vi "Fit and Plot Metric v2.vi"() -> (3 "Peak":dbl)   [LabVIEW 2014]
uses:
  <vilib>/Analysis/NI_AALPro.lvlib
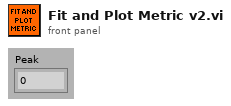
[diagram p1: front panel]
types:
  T1 = cluster{"Ab Corr VI.I":dbl[], "Ab Corr VI.I":dbl[]}
  T2 = cluster{"Ab Corr VI.I":dbl[], "Ab Corr VI.I":dbl[]}[]
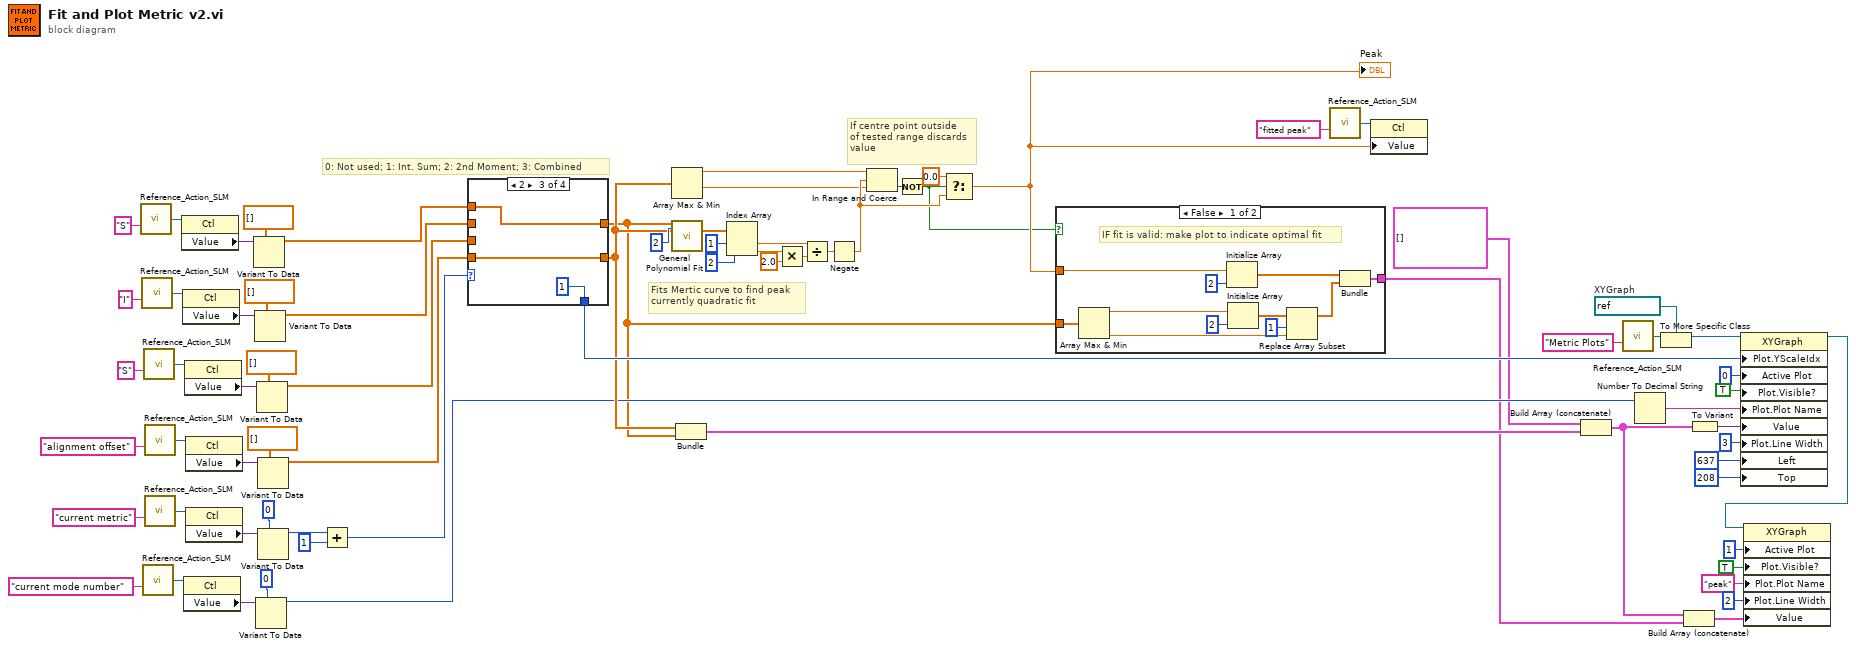
[diagram p0: block diagram]
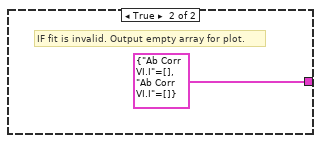
[diagram p2: hidden frame]
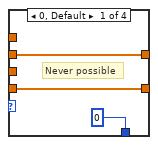
[diagram p3: hidden frame]
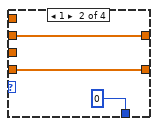
[diagram p4: hidden frame]
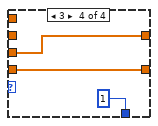
[diagram p5: hidden frame]
diagram:
  w26 = refnum<vi> refnum  # XYGraph
  # "0: Not used; 1: Int. Sum; 2: 2nd Moment; 3: Combined"
  # "Fits Mertic curve to find peak\ncurrently quadratic fit"
  # "If centre point outside \nof tested range discards\nvalue"
  n1 = call "Reference_Action_SLM.vi"("Control Name"="S") -> ("Ref OUT"=w54:refnum<vi>)  [unwired: 12 in, 2 out]
  n2 = call "Reference_Action_SLM.vi"("Control Name"="I") -> ("Ref OUT"=w49:refnum<vi>)  [unwired: 12 in, 2 out]
  n3 = call "Reference_Action_SLM.vi"("Control Name"="current mode number") -> ("Ref OUT"=w57:refnum<vi>)  [unwired: 12 in, 2 out]
  n4 = call "Reference_Action_SLM.vi"("Control Name"="S") -> ("Ref OUT"=w45:refnum<vi>)  [unwired: 12 in, 2 out]
  n5 = call "Reference_Action_SLM.vi"("Control Name"="alignment offset") -> ("Ref OUT"=w34:refnum<vi>)  [unwired: 12 in, 2 out]
  n6 = call "Reference_Action_SLM.vi"("Control Name"="current metric") -> ("Ref OUT"=w41:refnum<vi>)  [unwired: 12 in, 2 out]
  n7 = property class="Ctl"(reference=w54) -> ("Value"=w53:variant)  [unwired: 1 in, 2 out]
  n8 = property class="Ctl"(reference=w49) -> ("Value"=w48:variant)  [unwired: 1 in, 2 out]
  n9 = property class="Ctl"(reference=w57) -> ("Value"=w56:variant)  [unwired: 1 in, 2 out]
  n10 = property class="Ctl"(reference=w45) -> ("Value"=w44:variant)  [unwired: 1 in, 2 out]
  n11 = property class="Ctl"(reference=w34) -> ("Value"=w33:variant)  [unwired: 1 in, 2 out]
  n12 = property class="Ctl"(reference=w41) -> ("Value"=w40:variant)  [unwired: 1 in, 2 out]
  n13 = Variant To Data(type=dbl[] [] ("Ab Corr VI.I"), Variant=w53) -> (data=w38:dbl[])  [unwired: 1 in, 1 out]
  n14 = Variant To Data(type=dbl[] [] ("Ab Corr VI.I"), Variant=w48) -> (data=w37:dbl[])  [unwired: 1 in, 1 out]
  n15 = Variant To Data(type=0 ("disabled index (col)"), Variant=w56) -> (data=w30:i32)  [unwired: 1 in, 1 out]
  n16 = Variant To Data(type=dbl[] [] ("Ab Corr VI.I"), Variant=w44) -> (data=w36:dbl[])  [unwired: 1 in, 1 out]
  n17 = Variant To Data(type=dbl[] [] ("Ab Corr VI.I"), Variant=w33) -> (data=w31:dbl[])  [unwired: 1 in, 1 out]
  n18 = Variant To Data(type=0 ("disabled index (col)"), Variant=w40) -> (data=w22:i32)  [unwired: 1 in, 1 out]
  n19 = Add(x=w22, y=1) -> (x+y=w21:i32)
  n20 = case shown="2" w21 {
    tunnel: [0 ("polynomial order") 0 ("polynomial order") 1 ("polynomial order") 1 ("polynomial order")] -> w62
    tunnel: w36 -> [_ _ _ w85]
    tunnel: w37 -> [w76 w79 _ _]
    tunnel: w38 -> [_ _ w82 _]
    tunnel: [w76 w79 w82 w85] -> w11
    tunnel: w31 -> [w75 w78 w81 w84]
    tunnel: [w75 w78 w81 w84] -> w59
    frame 0, Default {
      # "Never possible"
    }
    frame 1 {
    }
    frame 2 {
    }
    frame 3 {
    }
  }
  n21 = Array Max & Min(array=w59) -> (max value=w61:dbl, min value=w60:dbl)  [unwired: 2 out]
  n22 = call <vilib>:"General Polynomial Fit.vi"("Y"=w11, "polynomial order"=2, "X"=w59) -> ("Polynomial Coefficients"=w72:dbl[])  [unwired: 9 in, 3 out]
  n23 = Bundle("Ab Corr VI.I"=w59, "Ab Corr VI.I"=w11) -> (w18:T1)  [unwired: 1 out]
  n24 = Index Array(array=w72, index #1=1 ("index"), index #2=2 ("index")) -> (element #1=w69:dbl, element #2=w68:dbl)
  n25 = Multiply(x=w68, y=2.0) -> (x*y=w66:dbl)
  n26 = Divide(x=w69, y=w66) -> (x/y=w67:dbl)
  n27 = Negate(x=w67) -> (-x=w64:dbl)
  n28 = In Range and Coerce(upper limit=w61, x=w64, lower limit=w60) -> (In Range?=w74:bool)  [unwired: 1 out]
  n29 = Not(x=w74) -> (.not. x?=w12:bool)
  n30 = Select(t=0.0 ("center"), s=w12, f=w64) -> (s? t:f=w19:dbl)
  "Peak" <- w19
  n31 = case shown="False" w12 {
    tunnel: w11 -> [w94 _]
    tunnel: w19 -> [w90 _]
    tunnel: [w89 T1 {"Ab Corr VI.I"=[], "Ab Corr VI.I"=[]} ("output cluster")] -> w1
    frame False {
      # "IF fit is valid: make plot to indicate optimal fit"
      n32 = Array Max & Min(array=w94) -> (max value=w88:dbl, min value=w87:dbl)  [unwired: 2 out]
      n33 = Initialize Array(w90, 2 ("dimension size")) -> (w96:dbl[])
      n34 = Initialize Array(w88, 2 ("dimension size")) -> (w93:dbl[])
      n35 = Replace Array Subset(array=w93, new element=w87, index=1) -> (w91:dbl[])
      n36 = Bundle(w96, w91) -> (w89:cluster{dbl[], dbl[]})  [unwired: 1 out]
    }
    frame True {
      # "IF fit is invalid. Output empty array for plot."
    }
  }
  n37 = call "Reference_Action_SLM.vi"("Control Name"="fitted peak") -> ("Ref OUT"=w27:refnum<vi>)  [unwired: 12 in, 2 out]
  n38 = property class="Ctl"(reference=w27, "Value"=w19) -> ()  [unwired: 1 in, 2 out]
  n39 = Build Array (concatenate)(cluster{"Coeff Steps":dbl[], "M":dbl[]}[] [] ("appended array"), w18) -> (w5:T2)
  n40 = call "Reference_Action_SLM.vi"("Control Name"="Metric Plots") -> ("Ref OUT"=w25:refnum<vi>)  [unwired: 12 in, 2 out]
  n41 = Number To Decimal String(number=w30) -> (decimal integer string=w15:string)  [unwired: 1 out]
  n42 = To More Specific Class(target class=w26, reference=w25) -> (specific class reference=w2:refnum<vi>)  [unwired: 1 in, 1 out]
  n43 = Build Array (concatenate)(w5, w1) -> (w6:T2)
  n44 = To Variant(anything=w5) -> (Variant=w14:variant)
  n45 = property on="Property Node" class="XYGraph"(reference=w2, "Plot.YScaleIdx"=w62, "Active Plot"=u32 0, "Plot.Visible?"=TRUE ("Plot.Visible"), "Plot.Plot Name"=w15, "Value"=w14, "Plot.Line Width"=u8 3, "Left"=637 ("Position:Left"), "Top"=208 ("Position:Top")) -> (reference out=w4:refnum<vi>)  [unwired: 1 in, 1 out]
  n46 = property on="Property Node" class="XYGraph"(reference=w4, "Active Plot"=u32 1, "Plot.Visible?"=TRUE ("Plot.Visible"), "Plot.Plot Name"="peak", "Plot.Line Width"=u8 2, "Value"=w6) -> ()  [unwired: 1 in, 2 out]
